vi "Get Single-Multiple Statistics Measurement.vi"(6 "Measurement Group Size":enum16{"Single", "Multiple"}(ring), 8 "error in (no error)":errorcluster, 11 "Oscilloscope in":refnum<class "Oscilloscope.lvclass">) -> (0 "error out":errorcluster, 2 "Multiple Statistics":T1(array[cluster]), 3 "Oscilloscope out":refnum<class "Oscilloscope.lvclass">)   [LabVIEW 2018, in "Oscilloscope.lvlib" / "Oscilloscope.lvclass"]
doc: "Use only after Overrides: Setup Single Statistics Measurement.vi or Setup Multiple Statistics Measurement..\n\nOverrides: Measure Statistics.vi and Measure Statistics (Multiple).vi accomplish the Setup and Get Statistics in one single VI."
uses:
  Oscilloscope.lvclass
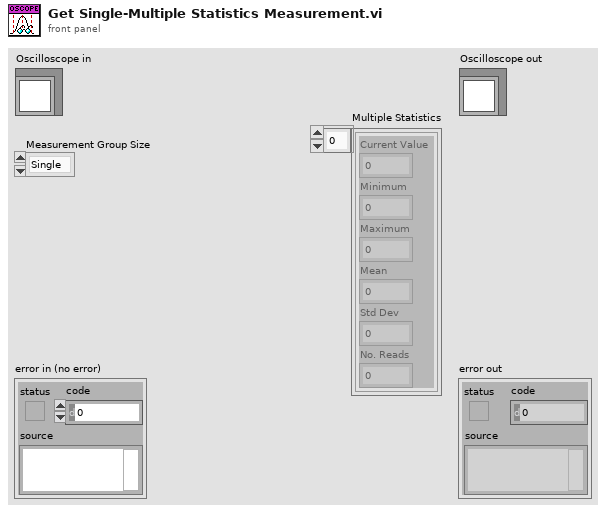
[diagram p1: front panel]
types:
  T1 = cluster{"Current Value":dbl, "Minimum":dbl, "Maximum":dbl, "Mean":dbl, "Std Dev":dbl, "No. Reads":dbl}[]
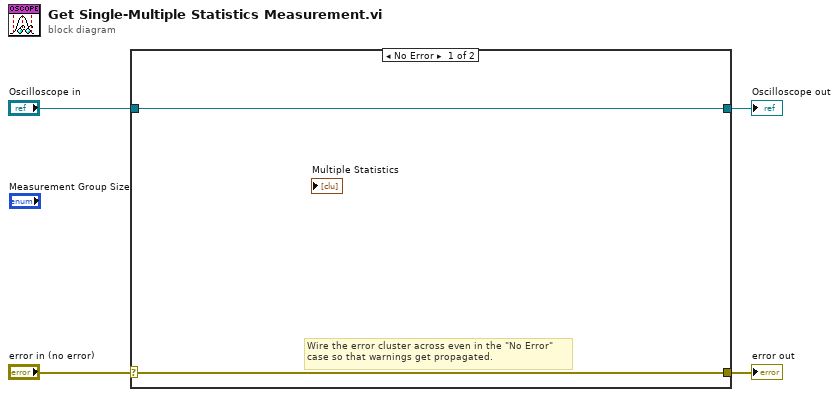
[diagram p0: block diagram]
diagram:
  n1 = case shown="No Error" "error in (no error)" {
    selector: "error in (no error)" -> [w5 w8]
    tunnel: [w5 w8] -> w3
    tunnel: [w6 w7] -> w1
    tunnel: "Oscilloscope in" -> [w6 w7]
    frame No Error {
      # "Wire the error cluster across even in the \"No Error\"\ncase so that warnings get propagated."
    }
    frame Error {
    }
  }
  "error out" <- w3
  "Oscilloscope out" <- w1
